vi "3NumToStr.vi"(1 "Num 3":i32, 2 "Num 2":i32, 3 "Num 1":i32) -> (0 "Combined Output String":string)   [LabVIEW 2013]
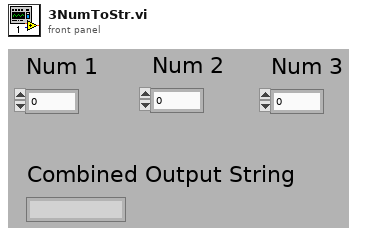
[diagram p1: front panel]
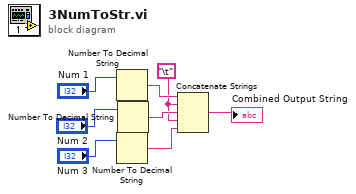
[diagram p0: block diagram]
diagram:
  w2 = "\t"
  n1 = Number To Decimal String(number="Num 1") -> (decimal integer string=w6:string)  [unwired: 1 in]
  n2 = Number To Decimal String(number="Num 3") -> (decimal integer string=w8:string)  [unwired: 1 in]
  n3 = Number To Decimal String(number="Num 2") -> (decimal integer string=w4:string)  [unwired: 1 in]
  n4 = Concatenate Strings(w6, w2, w4, w2, w8) -> (→"Combined Output String":string)
